vi "Disable Data Stream.vi"(8 "error in (no error)":errorcluster, 10 "req_stream_id":T1(ring)=enum."RAW_SENSORS", 11 "Aircraft ID":u8) -> (0 "error out":errorcluster)   [LabVIEW 2014]
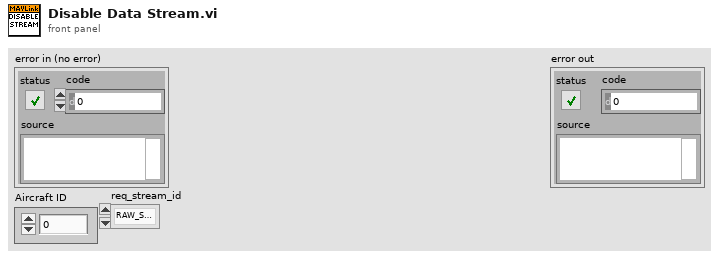
[diagram p1: front panel]
types:
  T1 = enum16{"ALL", "RAW_SENSORS", "EXTENDED_STATUS", "RC_CHANNELS", "RAW_CONTROLLER", "POSITION", "EXTRA1", "EXTRA2", "EXTRA3"}
  T2 = cluster{"req_message_rate":u16, "target_system":u8, "target_component":u8, "req_stream_id":enum16{"ALL", "RAW_SENSORS", "EXTENDED_STATUS", "RC_CHANNELS", "RAW_CONTROLLER", "POSITION", "EXTRA1", "EXTRA2", "EXTRA3"}, "start_stop":bool}
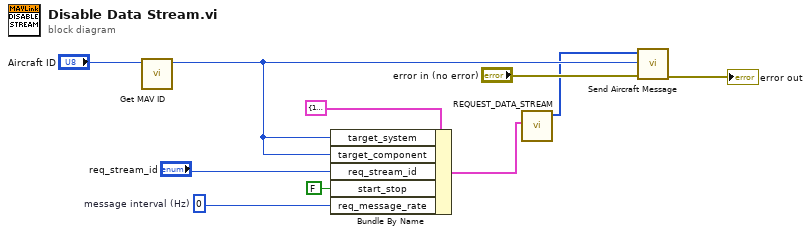
[diagram p0: block diagram]
diagram:
  w3 = u16 0  # message interval (Hz)
  n1 = call "Get MAV ID.vi"("Aircraft Index"="Aircraft ID") -> ("Aircraft ID"=w6:u8)  [unwired: 9 in, 1 out]
  n2 = Bundle By Name(cluster=T2 {"req_message_rate"=10, "target_system"=0, "target_component"=0, "req_stream_id"=enum."ALL", "start_stop"=FALSE} ("Payload"), "target_system"=w6, "target_component"=w6, "req_stream_id"="req_stream_id", "start_stop"=FALSE, "req_message_rate"=w3) -> (w2:T2)
  n3 = call "REQUEST_DATA_STREAM.vi"("Payload"=w2) -> ("MAVLink MSG"=w1:u8[])  [unwired: 10 in]
  n4 = call "Send Aircraft Message.vi"("error in (no error)"="error in (no error)", "Aircraft ID"=w6, "MAVLink Message"=w1) -> ("error out"=→"error out":errorcluster)  [unwired: 8 in]
